vi "sub_q-case_내구.vi"() -> ()   [LabVIEW 2019]
uses:
  _ctrl/create-rw-close.ctl
panel:
  in  "case":string
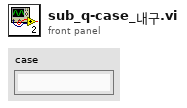
[diagram p1: front panel]
types:
  T1 = typedef "create-rw-close.ctl" = enum16{"create", "write", "read", "close"}
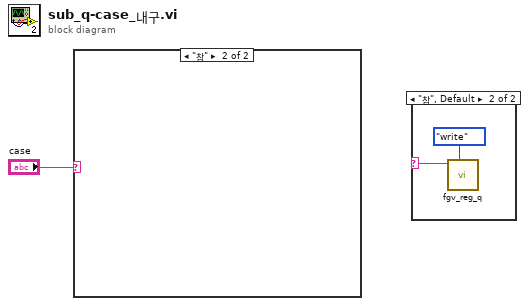
[diagram p0: block diagram]
diagram:
  n1 = case shown="\"참\"" "case" {
    frame "거짓", Default {
    }
    frame "참" {
    }
  }
  n2 = case shown="\"참\", Default" {
    selector: _ -> [_ w2]
    frame "" {
    }
    frame "참", Default {
      n3 = call "fgv_reg_q.vi"("cmd"=create-rw-close."write", "action"=w2) -> ()  [unwired: 8 in, 2 out]
    }
  }
